vi "1_Waveform_Signal_Regression_Multi_Output(Training).vi"() -> ()   [LabVIEW 2020]
uses:
  <vilib>/Ngene/Deep Learning Toolkit/Toolkit/NN_Train/Controls/NN_LR_Policy_Cfg.ctl
  <vilib>/Ngene/Deep Learning Toolkit/Toolkit/NN_Train/Controls/NN_LR_Policy_Type.ctl
  <vilib>/Ngene/Deep Learning Toolkit/Toolkit/NN_Train/Controls/NN_Train_Session_Data.ctl
  <vilib>/Ngene/Deep Learning Toolkit/Toolkit/NN_Train/Controls/NN_Train_Params.ctl
  <vilib>/Ngene/Deep Learning Toolkit/Toolkit/NN_Train/Controls/NN_Train_Optimizer.ctl
  <vilib>/Ngene/Deep Learning Toolkit/Toolkit/NN_Train/Controls/NN_Train_Data_Sampling.ctl
  <vilib>/Ngene/Deep Learning Toolkit/Toolkit/NN_Network/Controls/NN_Device.ctl
  <vilib>/Ngene/Deep Learning Toolkit/Toolkit/NN_Layers/Layers/Input/Controls/NN_Layer_Config(Input1D).ctl
  <vilib>/Ngene/Deep Learning Toolkit/Toolkit/NN_Data/Controls/NN_Data_type.ctl
  <vilib>/Ngene/Deep Learning Toolkit/Toolkit/NN_Layers/Layers/FC/Controls/NN_Layer_Config(FC).ctl
  <vilib>/Ngene/Deep Learning Toolkit/Toolkit/NN_Layers/Layers/BatchNorm/Controls/NN_BN_Params.ctl
  <vilib>/Ngene/Deep Learning Toolkit/Toolkit/NN_Activations/Controls/NN_Activation_Type.ctl
  <vilib>/Ngene/Deep Learning Toolkit/Toolkit/NN_Layers/Controls/NN_Layer_Init_Params.ctl
  <vilib>/Ngene/Deep Learning Toolkit/Toolkit/NN_Layers/Controls/NN_Layer_Weight_Init_Type.ctl
  <vilib>/Ngene/Deep Learning Toolkit/Toolkit/NN_Network/Controls/NN_Save_Before_Destroy_Options.ctl
  <vilib>/Ngene/Deep Learning Toolkit/Toolkit/NN_Layers/Layers/Input/NN_Layer_Create(Input1D).vi
  <vilib>/Ngene/Deep Learning Toolkit/Toolkit/NN_Layers/Layers/FC/NN_Layer_Create(FC).vi
  <vilib>/Ngene/Deep Learning Toolkit/Toolkit/NN_Train/Loss_Functions/NN_Set_Loss(MSE).vi
  <vilib>/Ngene/Deep Learning Toolkit/Toolkit/NN_Network/subVIs/NN_Predict/NN_Predict(In1D_Out1D).vi
  <vilib>/Ngene/Deep Learning Toolkit/Toolkit/NN_Train/Eval_Loss/NN_Eval_Test_Error_Loss/NN_Eval(In1D_Out1D).vi
  <vilib>/Ngene/Deep Learning Toolkit/Toolkit/Deep_Learning_Toolkit_by_Ngene.lvlib
  <vilib>/ptbypt/NI_PtbyPt.lvlib
panel:
  out "Training Loss":sgl=0.03699636 format="%#.6g"
  in  "Eval":bool
  out "Loss Graphs":cluster{"mean":dbl, "mean":dbl}(graph)={"mean"=0.04953590838238597, "mean"=0.07946349680423737}
  in  "NN_Device":T1=enum."GPU"
  out "Test Loss":sgl=0.0794635 format="%#.6g"
  in  "Stop Training":bool
  in  "NN_Train_Params":T2={"Optimizer"=enum."Adam", "Beta_1"=0.9, "Beta_2"=0.999, "Weight Decay(L1)"=1e-07, "Weight Decay(L2)"=1e-07, "Data_Sampling"=enum."Random"}
  out "Session Data":T5={"Epochs"=13.59232, "Tot_Iter"=10619, "LR"=0.00025, "LR_iter"=10620}
  in  "LR Update Policy":T6={"Policy_Type"=enum."Step", "LR0"=0.001, "k"=5.0, "WarmUp_Policy"=enum."Ramp", "WarmUp_Iter"=1000, "WarmUp_Ratio"=100.0} {"WarmUp_Ratio" min=1; "WarmUp_Iter" min=1; "LR0" format="%.7f"}
  # "Overview: This example demonstrates the usage of Deep Learning Toolkit for solving multiple output waveform signal regression problem. Specifically, a model is trained to predict multiple characteristic properties of a waveform, such as frequency, amplitude, phase, and DC offset..\nRequirements: DeepLTK - Deep Learning Toolkit for LabVIEW.\nInstructions:\n1.  Run the VI with current configuration of the training parameters and Learning Rate update policy.\n2. Observe how the training loss is decreasing.\n3. Press the \"Stop Training\" when the loss is not decreasing any more.\nMore Examples:  https://github.com/ngenehub/deepltk_examples"
  # "Waveform Signal Regression (Training)\nMultiple Property Prediction"
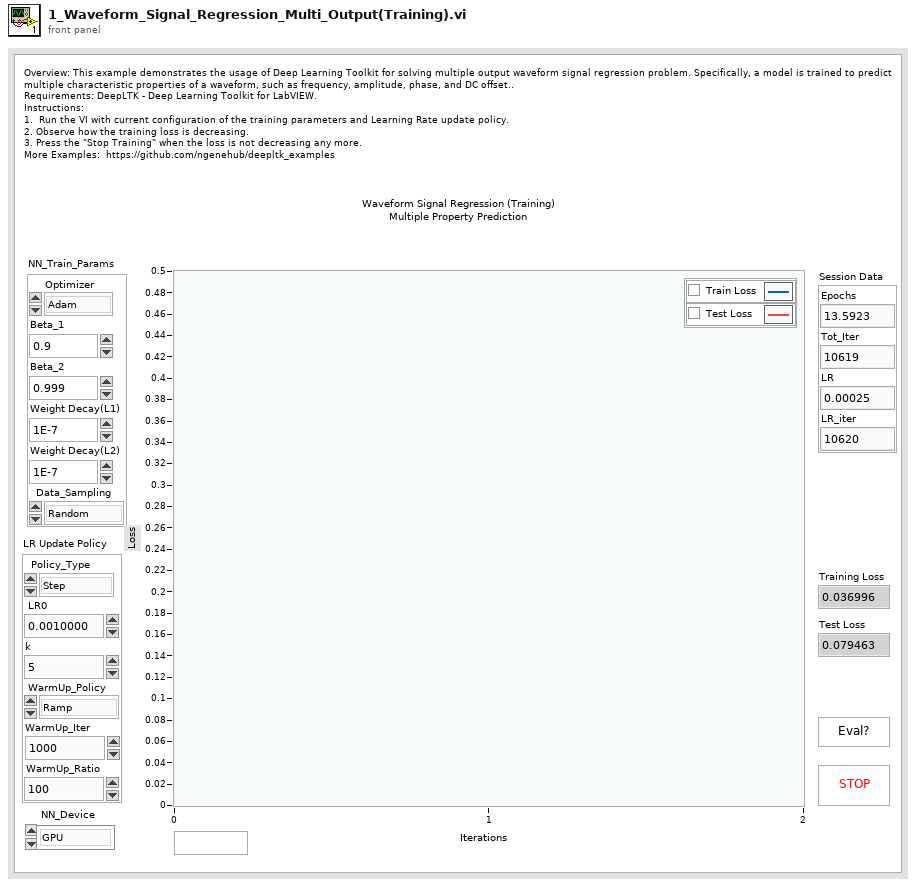
[diagram p1: front panel]
types:
  T1 = typedef "Deep_Learning_Toolkit_by_Ngene.lvlib/NN_Device.ctl" = enum16{"CPU", "GPU"}
  T2 = typedef "Deep_Learning_Toolkit_by_Ngene.lvlib/NN_Train_Params.ctl" = cluster{"Optimizer":T3, "Beta_1":sgl, "Beta_2":sgl, "Weight Decay(L1)":sgl, "Weight Decay(L2)":sgl, "Data_Sampling":T4}
  T3 = typedef "Deep_Learning_Toolkit_by_Ngene.lvlib/NN_Train_Optimizer.ctl" = enum16{"SGD", "Adam", "Adagrad", "Adadelta", "RMSProp", "Nesterov"}
  T4 = typedef "Deep_Learning_Toolkit_by_Ngene.lvlib/NN_Train_Data_Sampling.ctl" = enum16{"Random", "Sequential"}
  T5 = typedef "Deep_Learning_Toolkit_by_Ngene.lvlib/NN_Train_Session_Data.ctl" = cluster{"Epochs":sgl, "Tot_Iter":i32, "LR":sgl, "LR_iter":i32}
  T6 = typedef "Deep_Learning_Toolkit_by_Ngene.lvlib/NN_LR_Policy_Cfg.ctl" = cluster{"Policy_Type":T7, "LR0":dbl, "k":sgl, "WarmUp_Policy":enum16{"Step", "Ramp"}, "WarmUp_Iter":i32, "WarmUp_Ratio":sgl}
  T7 = typedef "Deep_Learning_Toolkit_by_Ngene.lvlib/NN_LR_Policy_Type.ctl" = enum16{"Manual", "Step", "Exp", "1/t"}
  T8 = typedef "Deep_Learning_Toolkit_by_Ngene.lvlib/NN_Layer_Config(FC).ctl" = cluster{"Name":string, "Size":i32, "BN":bool, "BN_Params":T9, "Activation":T10, "Has Bias?":bool, "Init_Params":T11, "Custom_Params":string}
  T9 = typedef "Deep_Learning_Toolkit_by_Ngene.lvlib/NN_BN_Params.ctl" = cluster{"epsilon":sgl, "momentum":sgl}
  T10 = typedef "Deep_Learning_Toolkit_by_Ngene.lvlib/NN_Activation_Type.ctl" = enum16{"Sigmoid", "ReLU", "LReLU", "ReLU6", "tanh", "Swish", "Mish", "None"}
  T11 = typedef "Deep_Learning_Toolkit_by_Ngene.lvlib/NN_Layer_Init_Params.ctl" = cluster{"Init_Type":T12, "Value":sgl}
  T12 = typedef "Deep_Learning_Toolkit_by_Ngene.lvlib/NN_Layer_Weight_Init_Type.ctl" = enum16{"Const", "Uniform", "Gaussian", "Xavier"}
  T13 = typedef "Deep_Learning_Toolkit_by_Ngene.lvlib/NN_Save_Before_Destroy_Options.ctl" = cluster{"CFG?":bool, "Weights?":bool, "Render?":bool}
  T14 = typedef "Deep_Learning_Toolkit_by_Ngene.lvlib/NN_Layer_Config(Input1D).ctl" = cluster{"Name":string, "Size":i32, "Data_Type":T15, "Shift":sgl, "Scale":sgl}
  T15 = typedef "Deep_Learning_Toolkit_by_Ngene.lvlib/NN_Data_type.ctl" = enum16{"I8", "U8", "I16", "U16", "U32 ARGB", "SGL"}
  T16 = typedef "Deep_Learning_Toolkit_by_Ngene.lvlib/NN_DataSets_All(In1D_Out1D).ctl" = cluster{"Train":T17, "Validation":T17, "Test":T17}
  T17 = typedef "Deep_Learning_Toolkit_by_Ngene.lvlib/NN_DataSet(In1D_Out1D).ctl" = cluster{"Inputs Ref.":variant, "Outputs Ref.":T18, "Dims_In":i32, "Dataset_Size":i32, "Dims_Out":i32, "Labels":string[], "File Paths":path[]}
  T18 = typedef "Deep_Learning_Toolkit_by_Ngene.lvlib/NN_Data_ref(2D_SGL).ctl" = refnum<data-value>
  T19 = typedef "Deep_Learning_Toolkit_by_Ngene.lvlib/NN.ctl" = cluster{"Name":string, "No of Layers":i32, "mBatch":i32, "Layers":T20[], "Dimty":T21, "Dims_In":T22, "Dims_Out":T22, "Working_Dir":path, "Train?":bool, "Train_Params":T2, "LR_Update_Policy":T6, "Session Data":T5, "Ground_truth":T23, "NNg_hdls":T24, "NN_Device":T1, "GPU Id":i32, "Labels":string[], "Receptive Field":T25[], "Loss_Type":T26, "Loss_Cfg_Prms":variant, "NNG_WS":T27}
  T20 = typedef "Deep_Learning_Toolkit_by_Ngene.lvlib/NN_Layer_ref.ctl" = refnum<data-value>
  T21 = typedef "Deep_Learning_Toolkit_by_Ngene.lvlib/NN_In_Out_Dim-ty.ctl" = enum8{"In1D_Out1D", "In3D_Out1D", "In3D_Out3D", "In3D_OutBBox"}
  T22 = typedef "Deep_Learning_Toolkit_by_Ngene.lvlib/NN_Dims(C,H,W).ctl" = cluster{"C":i32, "H":i32, "W":i32}
  T23 = typedef "Deep_Learning_Toolkit_by_Ngene.lvlib/NN_Ground_truth.ctl" = cluster{"Y":variant}
  T24 = typedef "Deep_Learning_Toolkit_by_Ngene.lvlib/nng_cuda_handles.ctl" = cluster{"cudnn":u64, "cublas":u64, "stream":u64, "curand":u64}
  T25 = typedef "Deep_Learning_Toolkit_by_Ngene.lvlib/NN_Dims(V,H).ctl" = cluster{"V":i32, "H":i32}
  T26 = typedef "Deep_Learning_Toolkit_by_Ngene.lvlib/NN_Loss_Type.ctl" = enum16{"None", "MSE", "CrossEntropy", "YOLO_v2", "YOLO_v4"}
  T27 = typedef "Deep_Learning_Toolkit_by_Ngene.lvlib/NNG_WS.ctl" = cluster{"NNG_WS_Mem":T28, "Max_WS_Size":i64}
  T28 = typedef "Deep_Learning_Toolkit_by_Ngene.lvlib/NNg_WS_Mem_DVR.ctl" = refnum<data-value>
  T29 = typedef "Deep_Learning_Toolkit_by_Ngene.lvlib/NN_Eval_Params.ctl" = cluster{"Loss":sgl, "Error":sgl}
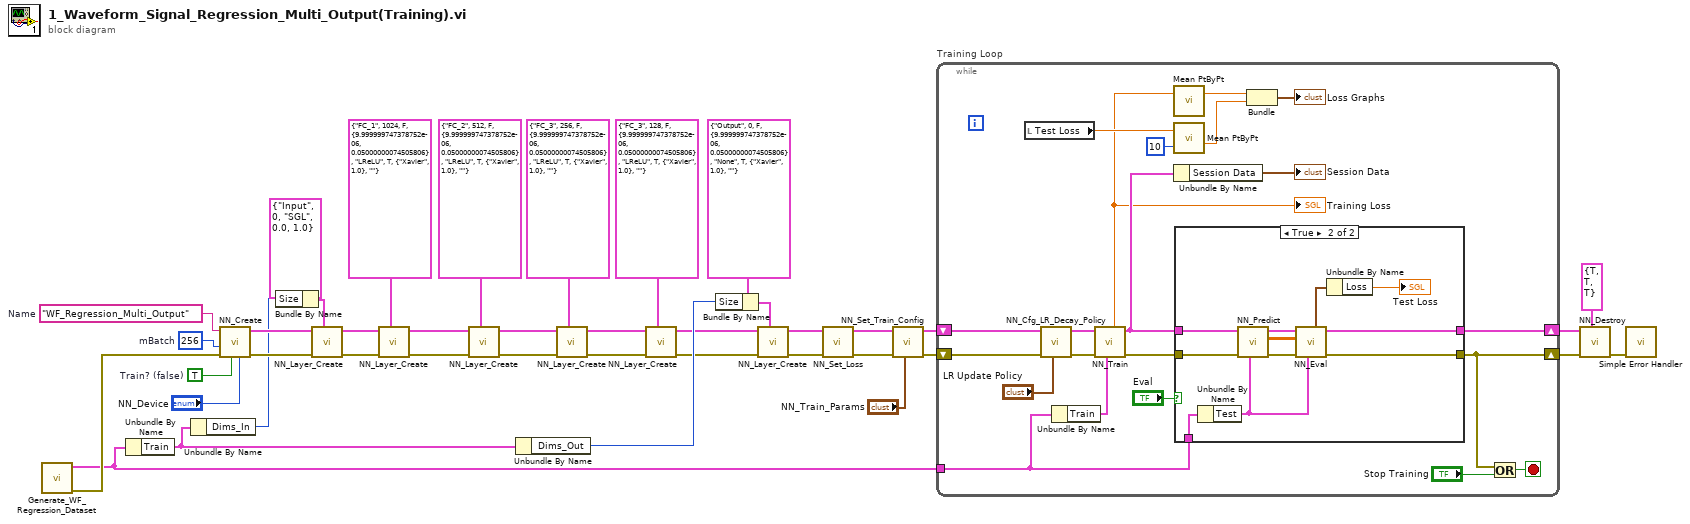
[diagram p0: block diagram]
diagram:
  w21 = "WF_Regression_Multi_Output"  # Name
  w22 = 256  # mBatch
  w23 = TRUE  # Train? (false)
  n1 = call "Generate_WF_Regression_Dataset.vi"() -> ("error out"=w32:errorcluster, "DataSets_All(In1D_Out1D)"=w8:T16)  [unwired: 10 in]
  n2 = Unbundle By Name(w8) -> ("Train"=w6:T17)
  n3 = Unbundle By Name(w6) -> ("Dims_In"=w30:i32)
  n4 = call <vilib>:"NN_Create.vi"("NN_Device"="NN_Device", "Train? (false)"=w23, "error in (no error)"=w32, "mBatch (1)"=w22, "Name"=w21) -> ("error out"=w39:errorcluster, "NN out"=w40:T19)  [unwired: 5 in]
  n5 = Bundle By Name(cluster=T14 {"Name"="Input", "Size"=0, "Data_Type"=enum."SGL", "Shift"=0.0, "Scale"=1.0} ("Input1D_Cfg"), "Size"=w30) -> (w31:T14)
  n6 = call-poly <vilib>:"NN_Layer_Create.vi"("Input1D_Cfg"=w31, "error in (no error)"=w39, "NN in"=w40) -> ("error out"=w26:errorcluster, "NN out"=w27:T19)  [unwired: 6 in, 1 out]
  n7 = call-poly <vilib>:"NN_Layer_Create.vi"("FC_Cfg"=T8 {"Name"="FC_1", "Size"=1024, "BN"=FALSE, "BN_Params"={"epsilon"=1e-05, "momentum"=0.05}, "Activation"=enum."LReLU", "Has Bias?"=TRUE, "Init_Params"={"Init_Type"=enum."Xavier", "Value"=1.0}, "Custom_Params"=""} ("FC_Cfg_1"), "error in (no error)"=w26, "NN in"=w27) -> ("error out"=w15:errorcluster, "NN out"=w16:T19)  [unwired: 6 in, 1 out]
  n8 = call-poly <vilib>:"NN_Layer_Create.vi"("FC_Cfg"=T8 {"Name"="FC_2", "Size"=512, "BN"=FALSE, "BN_Params"={"epsilon"=1e-05, "momentum"=0.05}, "Activation"=enum."LReLU", "Has Bias?"=TRUE, "Init_Params"={"Init_Type"=enum."Xavier", "Value"=1.0}, "Custom_Params"=""} ("FC_Cfg_1"), "error in (no error)"=w15, "NN in"=w16) -> ("error out"=w11:errorcluster, "NN out"=w12:T19)  [unwired: 6 in, 1 out]
  n9 = Unbundle By Name(w6) -> ("Dims_Out"=w28:i32)
  n10 = call-poly <vilib>:"NN_Layer_Create.vi"("FC_Cfg"=T8 {"Name"="FC_3", "Size"=256, "BN"=FALSE, "BN_Params"={"epsilon"=1e-05, "momentum"=0.05}, "Activation"=enum."LReLU", "Has Bias?"=TRUE, "Init_Params"={"Init_Type"=enum."Xavier", "Value"=1.0}, "Custom_Params"=""} ("FC_Cfg_1"), "error in (no error)"=w11, "NN in"=w12) -> ("error out"=w3:errorcluster, "NN out"=w4:T19)  [unwired: 6 in, 1 out]
  n11 = call-poly <vilib>:"NN_Layer_Create.vi"("FC_Cfg"=T8 {"Name"="FC_3", "Size"=128, "BN"=FALSE, "BN_Params"={"epsilon"=1e-05, "momentum"=0.05}, "Activation"=enum."LReLU", "Has Bias?"=TRUE, "Init_Params"={"Init_Type"=enum."Xavier", "Value"=1.0}, "Custom_Params"=""} ("FC_Cfg_1"), "error in (no error)"=w3, "NN in"=w4) -> ("error out"=w1:errorcluster, "NN out"=w2:T19)  [unwired: 6 in, 1 out]
  n12 = Bundle By Name(cluster=T8 {"Name"="Output", "Size"=0, "BN"=FALSE, "BN_Params"={"epsilon"=1e-05, "momentum"=0.05}, "Activation"=enum."None", "Has Bias?"=TRUE, "Init_Params"={"Init_Type"=enum."Xavier", "Value"=1.0}, "Custom_Params"=""} ("FC_Cfg_1"), "Size"=w28) -> (w29:T8)
  n13 = call-poly <vilib>:"NN_Layer_Create.vi"("FC_Cfg"=w29, "error in (no error)"=w1, "NN in"=w2) -> ("error out"=w35:errorcluster, "NN out"=w36:T19)  [unwired: 6 in, 1 out]
  n14 = call-poly <vilib>:"NN_Set_Loss.vi"("error in (no error)"=w35, "NN in"=w36) -> ("error out"=w18:errorcluster, "NN out"=w19:T19)  [unwired: 8 in]
  n15 = call <vilib>:"NN_Set_Train_Config.vi"("NN_Train_Params"="NN_Train_Params", "error in (no error)"=w18, "NN in"=w19) -> ("error out"=w24:errorcluster, "NN out"=w25:T19)  [unwired: 7 in]
  n16 = while "Training Loop" {
    shift-right: [w46] -> w9
    shift-left: w24 -> [w56]
    shift-right: [w52] -> w10
    shift-left: w25 -> [w59]
    tunnel: w8 -> [w42]
    stop <- w47 stop-if-true
    n17 = local read "Test Loss"() -> (w50:sgl)
    n18 = call <vilib>:"NN_Cfg_LR_Decay_Policy.vi"("LR_Decay_Params"="LR Update Policy", "error in (no error)"=w56, "NN in"=w59) -> ("error out"=w57:errorcluster, "NN out"=w58:T19)  [unwired: 7 in]
    n19 = Unbundle By Name(w42) -> ("Train"=w41:T17)
    n20 = call <vilib>:"NN_Train.vi"("Train Dataset"=w41, "error in (no error)"=w57, "NN in"=w58) -> ("error out"=w53:errorcluster, "NN out"=w54:T19, "Loss"=w48:sgl)  [unwired: 3 in, 3 out]
    "Training Loss" <- w48
    n21 = call <vilib>:"Mean PtByPt.vi"("x"=w48) -> ("mean"=w44:dbl)  [unwired: 3 in, 1 out]
    n22 = call <vilib>:"Mean PtByPt.vi"("x"=w50, "sample length"=10) -> ("mean"=w45:dbl)  [unwired: 2 in, 1 out]
    n23 = Unbundle By Name(w54) -> ("Session Data"=→"Session Data":T5)
    n24 = case shown="True" "Eval" {
      tunnel: w54 -> [w63 w73]
      tunnel: w53 -> [w62 w72]
      tunnel: [w63 w71] -> w52
      tunnel: [w62 w68] -> w46
      tunnel: w42 -> [_ w67]
      frame False {
      }
      frame True {
        n25 = Unbundle By Name(w67) -> ("Test"=w66:T17)
        n26 = call-poly <vilib>:"NN_Predict.vi"("Dataset"=w66, "error in (no error)"=w72, "NN in"=w73) -> ("error out"=w74:errorcluster, "Predictions"=w69:sgl[][], "NN out"=w70:T19)  [unwired: 6 in]
        n27 = call-poly <vilib>:"NN_Eval.vi"("Dataset"=w66, "error in (no error)"=w74, "Predictions"=w69, "NN in"=w70) -> ("error out"=w68:errorcluster, "NN out"=w71:T19, "NN_Eval_Params"=w65:T29)  [unwired: 4 in, 1 out]
        n28 = Unbundle By Name(w65) -> ("Loss"=→"Test Loss":sgl)
      }
    }
    n29 = Bundle("mean"=w44, "mean"=w45) -> (→"Loss Graphs":cluster{"mean":dbl, "mean":dbl})  [unwired: 1 in]
    n30 = Or(x=w46, y="Stop Training") -> (x .or. y?=w47:bool)
  }
  n31 = call <vilib>:"NN_Destroy.vi"("Save (T, T, T)"=T13 {"CFG?"=TRUE, "Weights?"=TRUE, "Render?"=TRUE}, "error in (no error)"=w9, "NN in"=w10) -> ("error out"=w34:errorcluster)  [unwired: 7 in, 1 out]
  n32 = call <vilib>:"Simple Error Handler.vi"("error in (no error)"=w34) -> ()  [unwired: 4 in, 5 out]
